vi "IPCore.Name.GetGroup.vi"(11 "Name":string) -> (3 "Group":string)   [LabVIEW 2015, in "Fuel Injector Analysis Addon System Explorer.lvlib"]
uses:
  Fuel Injector Analysis Addon System Explorer.lvlib
  Shared/Constants.vi
  Shared/Fuel Injector Analysis Addon Shared.lvlib
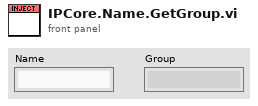
[diagram p1: front panel]
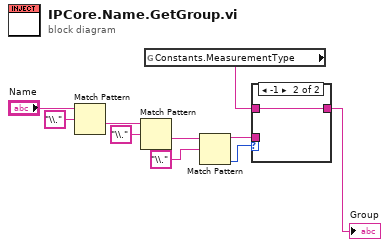
[diagram p0: block diagram]
diagram:
  n1 = Match Pattern(string="Name", regular expression="\\.") -> (after substring=w3:string)  [unwired: 1 in, 3 out]
  n2 = Match Pattern(string=w3, regular expression="\\.") -> (after substring=w5:string)  [unwired: 1 in, 3 out]
  n3 = global read "Constants.vi" "Constants.MeasurementType"() -> (w8:string)
  n4 = Match Pattern(string=w5, regular expression="\\.") -> (before substring=w9:string, offset past match=w7:i32)  [unwired: 1 in, 2 out]
  n5 = case shown="-1" w7 {
    tunnel: w8 -> [_ w12]
    tunnel: [w11 w12] -> w10
    tunnel: w9 -> [w11 _]
    frame Default {
    }
    frame -1 {
    }
  }
  "Group" <- w10
